vi "Main (9).vi"() -> ()   [LabVIEW 2016]
panel:
  out "LLenado":bool
  out "LLenado":bool
  out "Luz Baja 2":bool
  out "Luz Alta 2":bool
  in  "Dias Luz":string(combo)
  out "Unidades":string
  in  "Dias Temperatura":string(combo)
  in  "Centigrados":bool
  out "Intensidad  de Luz":u8(slide) scale=0.0..100.0
  out "Agua":dbl(slide) scale=0.0..200.0
  out "Comida":dbl(slide) scale=0.0..200.0
  out "Luz Baja":bool
  out "Luz Alta":bool
  out "Humedad":dbl(knob) scale=0.0..10.0
  out "H Baja":bool
  out "H Alta":bool
  out "T Baja":bool
  out "T Alta":bool
  out "Temperatura":dbl(slide) scale=0.0..100.0
  # "Granja de Pollitos\nMonitor de condiciones para una granja de pollitos"
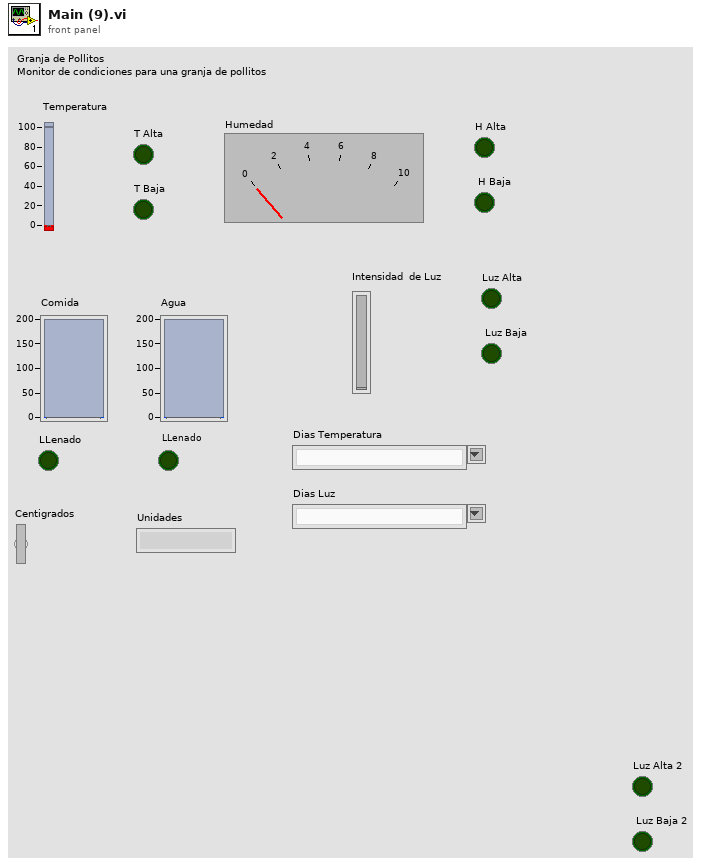
[diagram p1: front panel]
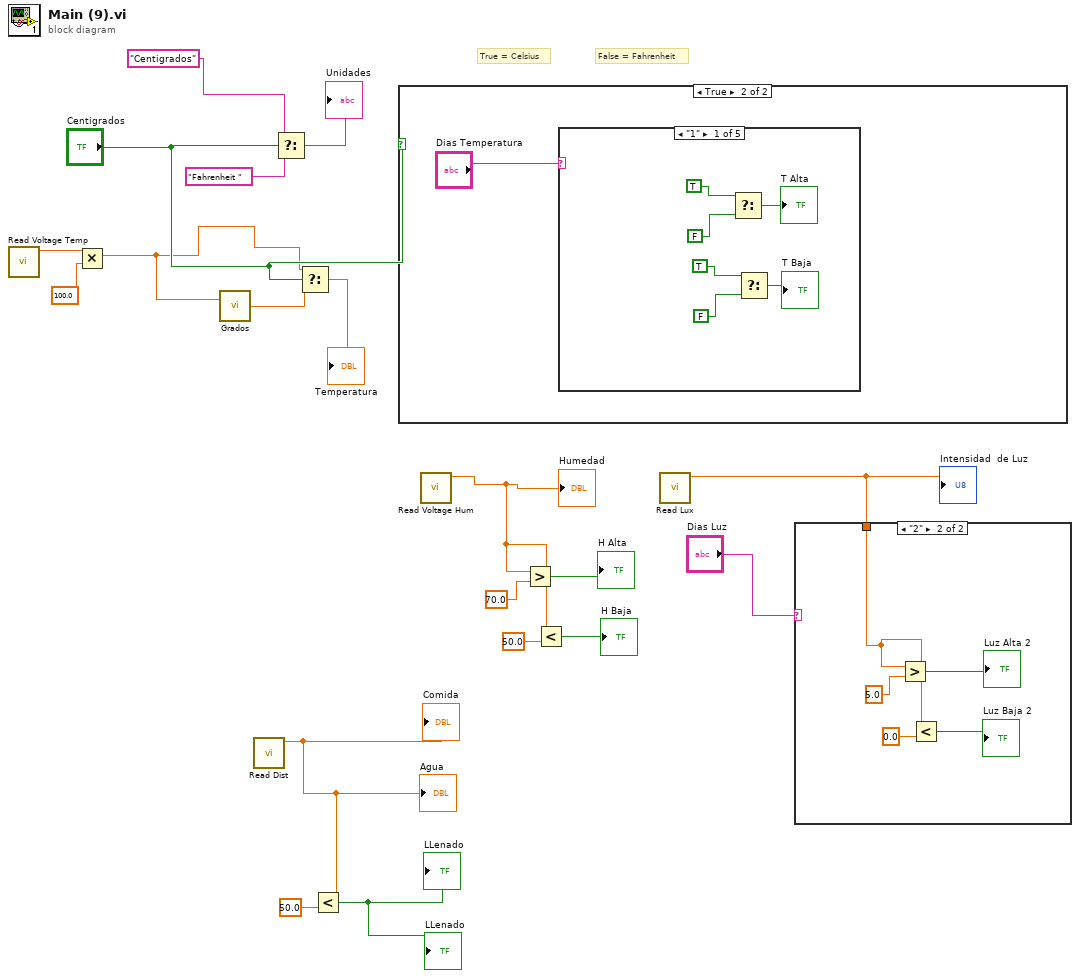
[diagram p0: block diagram]
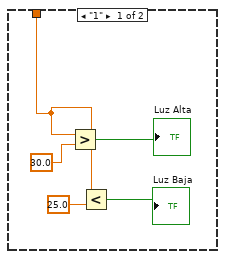
[diagram p2: hidden frame]
diagram:
  # "False = Fahrenheit"
  # "True = Celsius"
  n1 = call "Read Voltage Temp.vi"() -> ("Voltaje"=w14:dbl)  [unwired: 8 in, 1 out]
  n2 = Multiply(x=w14, y=100.0) -> (x*y=w12:dbl)
  n3 = call "Grados.vi"("Grado"=w12) -> ("Conversion"=w16:dbl)  [unwired: 1 in]
  n4 = call "Read Dist.vi"() -> ("distancia"=w3:dbl)  [unwired: 8 in, 1 out]
  "Comida" <- w3
  "Agua" <- w3
  n5 = Select(t="Centigrados", s="Centigrados", f="Fahrenheit ") -> (s? t:f=→"Unidades":string)
  n6 = Select(t=w12, s="Centigrados", f=w16) -> (s? t:f=→"Temperatura":dbl)
  n7 = Less?(x=w3, y=50.0) -> (x < y?=→"LLenado" →"LLenado":bool)
  n8 = case shown="True" "Centigrados" {
    frame False {
    }
    frame True {
      n9 = case shown="\"1\"" "Dias Temperatura" {
        frame "1" {
          n10 = Select(t=TRUE, f=FALSE) -> (s? t:f=→"T Alta":bool)  [unwired: 1 in]
          n11 = Select(t=TRUE, f=FALSE) -> (s? t:f=→"T Baja":bool)  [unwired: 1 in]
        }
        frame "2" {
        }
        frame "3" {
        }
        frame "4" {
        }
        frame "5" {
        }
      }
    }
  }
  n12 = call "Read Voltage Hum.vi"() -> ("Porcentaje"=w7:dbl)  [unwired: 8 in, 1 out]
  "Humedad" <- w7
  n13 = Greater?(x=w7, y=70.0) -> (0:→"H Alta":bool)
  n14 = Less?(x=w7, y=50.0) -> (x < y?=→"H Baja":bool)
  n15 = call "Read Lux.vi"() -> ("lux"=w5:dbl)  [unwired: 8 in, 1 out]
  "Intensidad  de Luz" <- w5
  n16 = case shown="\"2\"" "Dias Luz" {
    tunnel: w5 -> [w29 w32]
    frame "1" {
      n17 = Greater?(x=w29, y=30.0) -> (0:→"Luz Alta":bool)
      n18 = Less?(x=w29, y=25.0) -> (x < y?=→"Luz Baja":bool)
    }
    frame "2" {
      n19 = Greater?(x=w32, y=5.0) -> (0:→"Luz Alta 2":bool)
      n20 = Less?(x=w32, y=0.0) -> (x < y?=→"Luz Baja 2":bool)
    }
  }
